vi "CO MFR sw 2.vi"(8 "Increment":dbl, 9 "Bottle conc":dbl, 10 "C_CO":dbl, 11 "Flow rate":dbl) -> (3 "CO MFR":dbl)   [LabVIEW 2014]
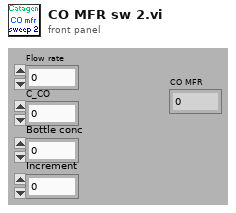
[diagram p1: front panel]
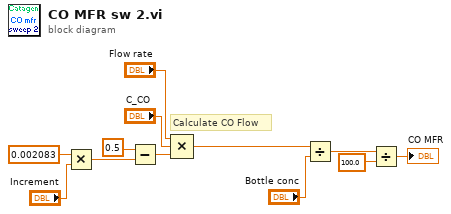
[diagram p0: block diagram]
diagram:
  # "Calculate CO Flow"
  n1 = Multiply(x=0.002083, y="Increment") -> (x*y=w4:dbl)
  n2 = Subtract(x=0.5, y=w4) -> (x-y=w1:dbl)
  n3 = Compound Arithmetic op=MULTIPLY("Flow rate", "C_CO", w1) -> (w8:dbl)
  n4 = Divide(x=w8, y="Bottle conc") -> (x/y=w7:dbl)
  n5 = Divide(x=w7, y=100.0) -> (x/y=→"CO MFR":dbl)
